vi "StartTrial.vi"(8 "error in (no error)":errorcluster, 11 "TrialBasedExperiment in":refnum<class "MatlabExperiment.lvclass">) -> (0 "error out":errorcluster, 3 "TrialBasedExperiment out":refnum<class "MatlabExperiment.lvclass">)   [LabVIEW 2010, in "MatlabExperiment.lvclass"]
uses:
  MatlabExperiment.lvclass
  TrialBasedExperimentObject/TrialBasedExperiment.lvclass
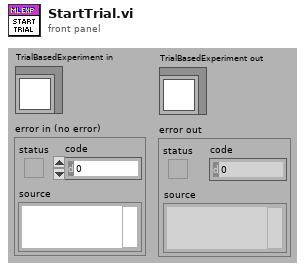
[diagram p1: front panel]
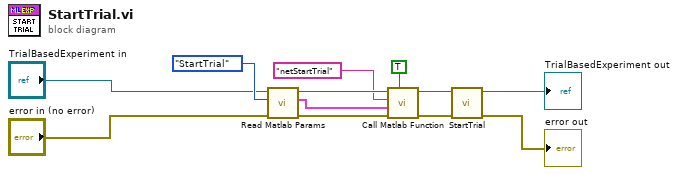
[diagram p0: block diagram]
diagram:
  n1 = call-dynamic "Read Matlab Params.vi"("error in (no error)"="error in (no error)", "Enum"=enum16{"StartSession", "StartTrial"}."StartTrial", "TrialBasedExperiment in"="TrialBasedExperiment in") -> ("error out"=w10:errorcluster, "Matlab Param Array"=w1:cluster{"Name":string, "Data":variant}[], "TrialBasedExperiment out"=w11:refnum<class "MatlabExperiment.lvclass">)  [unwired: 6 in]
  n2 = call-dynamic "Call Matlab Function.vi"("Timestamp"=TRUE, "error in (no error)"=w10, "Matlab Param Array"=w1, "Function name"="netStartTrial", "TrialBasedExperiment in"=w11) -> ("error out"=w7:errorcluster, "TrialBasedExperiment out"=w8:refnum<class "MatlabExperiment.lvclass">)  [unwired: 3 in, 2 out]
  n3 = call-parent "StartTrial.vi"("error in (no error)"=w7, "TrialBasedExperiment in"=w8) -> ("error out"=→"error out":errorcluster, "TrialBasedExperiment out"=→"TrialBasedExperiment out":refnum<class "MatlabExperiment.lvclass">)  [unwired: 8 in]
